vi "DDS Output Enable.vi"(8 "error in (no error)":errorcluster, 10 "enable":i32, 11 "channel_index":u8) -> (0 "error out":errorcluster)   [LabVIEW 2023, in "vmmsolib.lvlib"]
doc: "DLL_API void WINAPI DDSOutputEnable(unsigned char channel_index, int enable);"
uses:
  vmmsolib.lvlib
  vmmso.dll
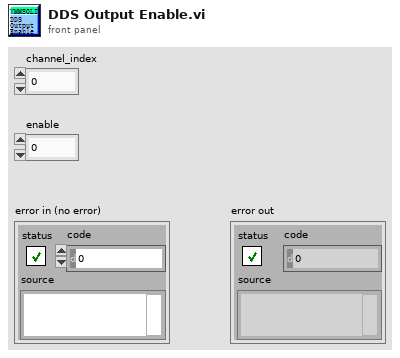
[diagram p1: front panel]
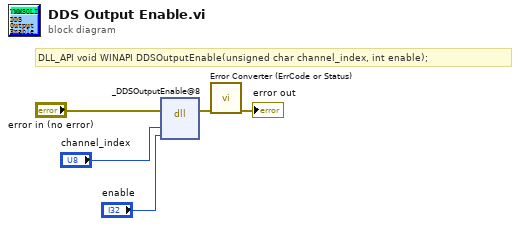
[diagram p0: block diagram]
diagram:
  # "DLL_API void WINAPI DDSOutputEnable(unsigned char channel_index, int enable);"
  n1 = dll-call lib="D:/VmMsoSDK/demo-Labview/2023/vmmsolib/vmmso.*" fn="_DDSOutputEnable@8"(error in="error in (no error)", "channel_index"="channel_index", "enable"="enable") -> (error out=w2:errorcluster)  [unwired: 5 in, 1 out]
  n2 = call "Error Converter (ErrCode or Status).vi"("error in (no error)"=w2) -> ("error out"=→"error out":errorcluster)  [unwired: 10 in]
